vi "Database-WriteDataToFile.vi"(8 "error in":errorcluster, 10 "Data":T1 {"Values" format="%.3f"}, 11 "Idx":i32) -> (0 "error out":errorcluster, 2 "Saved":bool)   [LabVIEW 2016]
doc: "Go to DB->WriteStationValues action\nReturn boolean flag to show if data was saved to DB successfully\n\nWabco 2017 All right reserved\nAuthor: maciej.szupienko@wabco-auto.com"
uses:
  Drivers/PLC/LowLevel/PLC.DataBlock.PLCvalues.ctl
  Database.Action.ctl
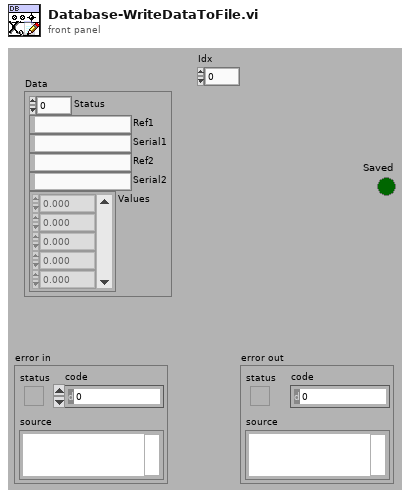
[diagram p1: front panel]
types:
  T1 = typedef "PLC.DataBlock.PLCvalues.ctl" = cluster{"Status":u8, "Ref1":string, "Serial1":string, "Ref2":string, "Serial2":string, "Values":sgl[]}
  T2 = typedef "Database.Action.ctl" = enum32{"idle", "constructor", "destructor", "--- DB ---", "Init", "Setup", "Changeover", "ExportData", "NewData", "GetPrevStatus", "CheckExist", "GetProdComp", "AddProdComp"}
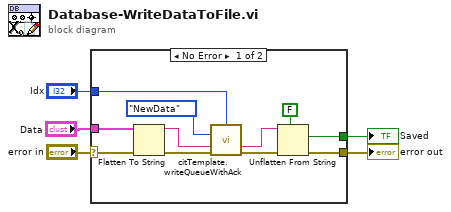
[diagram p0: block diagram]
diagram:
  n1 = case shown="No Error" "error in" {
    selector: "error in" -> [w16 w17]
    tunnel: [w11 w17] -> w4
    tunnel: "Data" -> [w15 _]
    tunnel: [w7 _] -> w3
    tunnel: "Idx" -> [w6 _]
    frame No Error {
      n2 = Flatten To String(anything=w15, error in (no error)=w16) -> (data string=w13:string, error out=w14:errorcluster)  [unwired: 2 in, 1 out]
      n3 = call "citTemplate.writeQueueWithAck.vi"("instance (0)"=w6, "event in"=Database.Action."NewData" ("Action"), "(flatten) data in"=w13, "error in (no error)"=w14) -> ("notification data"=w10:string, "error out"=w12:errorcluster)  [unwired: 9 in, 1 out]
      n4 = Unflatten From String(type=FALSE, binary string=w10, error in (no error)=w12) -> (value=w7:bool, error out=w11:errorcluster)  [unwired: 2 in, 1 out]
    }
    frame Error {
    }
  }
  "error out" <- w4
  "Saved" <- w3
